vi "IFA300HeaderList.vi"() -> (3 "appended array":string[](array[string]))   [LabVIEW 2011]
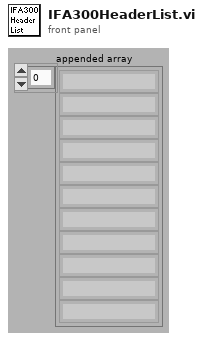
[diagram p1: front panel]
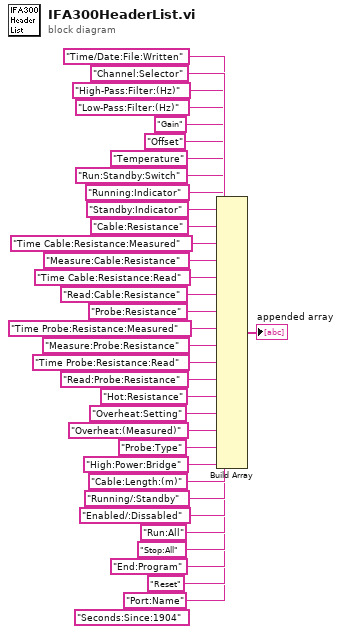
[diagram p0: block diagram]
diagram:
  n1 = Build Array("Time/Date:File:Written", "Channel:Selector", "High-Pass:Filter:(Hz)", "Low-Pass:Filter:(Hz)", "Gain", "Offset", "Temperature", "Run:Standby:Switch", "Running:Indicator", "Standby:Indicator", "Cable:Resistance", "Time Cable:Resistance:Measured", "Measure:Cable:Resistance", "Time Cable:Resistance:Read", "Read:Cable:Resistance", "Probe:Resistance", "Time Probe:Resistance:Measured", "Measure:Probe:Resistance", "Time Probe:Resistance:Read", "Read:Probe:Resistance", "Hot:Resistance", "Overheat:Setting", "Overheat:(Measured)", "Probe:Type", "High:Power:Bridge", "Cable:Length:(m)", "Running/:Standby", "Enabled/:Dissabled", "Run:All", "Stop:All", "End:Program", "Reset", "Port:Name", "Seconds:Since:1904") -> (→"appended array":string[])
